vi "Mutate 1.1.1.vi"(8 "error in (no error)":errorcluster, 11 "Device Ref in":T1 format="%.0x") -> (0 "error out":errorcluster, 3 "Device Ref out":T1 format="%.0x")   [LabVIEW 2020, in "Engine Simulation Toolkit System Explorer.lvlib"]
uses:
  Engine Simulation Toolkit System Explorer.lvlib
  <vilib>/NI VeriStand/Custom Device API/Custom Device Item Ref.ctl
  Shared/Properties.vi
  <vilib>/NI VeriStand/Custom Device API/Get Item Property (String).vi
  <vilib>/NI VeriStand/Custom Device API/Set Item Property (String).vi
  Shared/Engine Simulation Toolkit Shared.lvlib
  <vilib>/NI VeriStand/Custom Device API/Custom Device API.lvlib
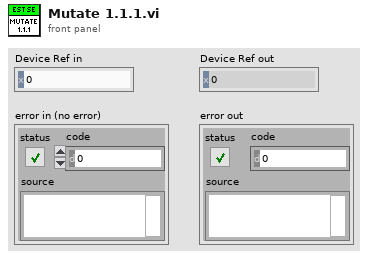
[diagram p1: front panel]
types:
  T1 = typedef "Custom Device API.lvlib/Custom Device Item Ref.ctl" = u64
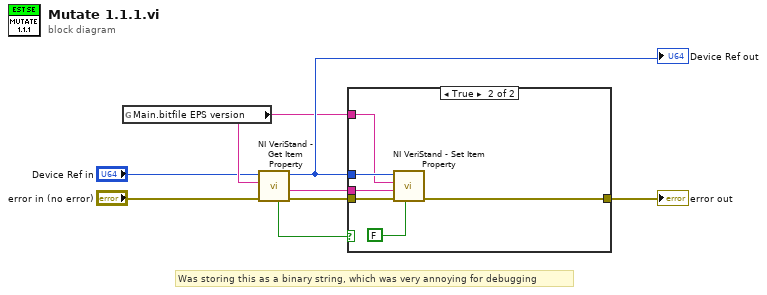
[diagram p0: block diagram]
diagram:
  # "Was storing this as a binary string, which was very annoying for debugging"
  n1 = global read "Properties.vi" "Main.bitfile EPS version"() -> (w5:string)
  n2 = call-poly <vilib>:"NI VeriStand - Get Item Property.vi"("error in (no error)"="error in (no error)", "Property Name"=w5, "Item Ref in"="Device Ref in") -> ("error out"=w4:errorcluster, "Value"=w6:string, "Item Ref out"=w8:T1, "Found?"=w3:bool)  [unwired: 5 in]
  "Device Ref out" <- w8
  n3 = case shown="True" w3 {
    tunnel: w8 -> [_ w15]
    tunnel: w4 -> [w9 w14]
    tunnel: w5 -> [_ w13]
    tunnel: w6 -> [_ w12]
    tunnel: [w9 w10] -> w7
    frame False {
    }
    frame True {
      n4 = call-poly <vilib>:"NI VeriStand - Set Item Property.vi"("Binary String (T)"=FALSE, "error in (no error)"=w14, "Value"=w12, "Property Name"=w13, "Item Ref in"=w15) -> ("error out"=w10:errorcluster)  [unwired: 4 in, 2 out]
    }
  }
  "error out" <- w7
